vi "Deadzone.vi"(1 "DeadZone":dbl, 2 "In":dbl) -> (0 "Out":dbl)   [LabVIEW 2018]
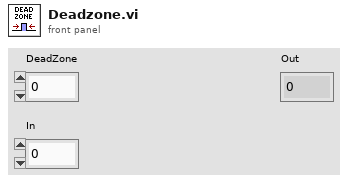
[diagram p1: front panel]
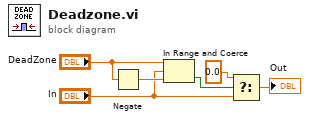
[diagram p0: block diagram]
diagram:
  n1 = Negate(x="DeadZone") -> (-x=w2:dbl)
  n2 = In Range and Coerce(upper limit="DeadZone", x="In", lower limit=w2) -> (In Range?=w4:bool)  [unwired: 1 out]
  n3 = Select(t=0.0, s=w4, f="In") -> (s? t:f=→"Out":dbl)
